vi "RT Acquisition and Logging.vi"(8 "error in (no error)":errorcluster, 10 "info":cluster{"File path":T4, "Cfg ":T5} {"Cfg"."Offset_rueda WS 2" format="%.27g"; "Cfg"."Offset_rueda WS 1" format="%.27g"; "Cfg"."Frecuencia de muestreo y módulo CRIO" items=["51.200 kS/s (NI 9234)"=1, "25.600 kS/s (NI 9234)"=2, "17.067 kS/s (NI 9234)"=3, "12.800 kS/s (NI 9234)"=4, "10.240 kS/s (NI 9234)"=5, "8.533 kS/s (NI 9234)"=6, "7.314 kS/s (NI 9234)"=7, "6.400 kS/s (NI 9234)"=8, "5.689 kS/s (NI 9234)"=9, "5.120 kS/s (NI 9234)"=10, "4.654 kS/s (NI 9234)"=11, "4.267 kS/s (NI 9234)"=12, "3.938 kS/s (NI 9234)"=13, "3.657 kS/s (NI 9234)"=14, "3.413 kS/s (NI 9234)"=15, "3.200 kS/s (NI 9234)"=16, "3.012 kS/s (NI 9234)"=17, "2.845 kS/s (NI 9234)"=18, "2.695 kS/s (NI 9234)"=19, "2.560 kS/s (NI 9234)"=20, "2.438 kS/s (NI 9234)"=21, "2.328 kS/s (NI 9234)"=22, "2.226 kS/s (NI 9234)"=23, "2.133 kS/s (NI 9234)"=24, "2.048 kS/s (NI 9234)"=25, "1.969 kS/s (NI 9234)"=26, "1.896 kS/s (NI 9234)"=27, "1.829 kS/s (NI 9234)"=28, "1.765 kS/s (NI 9234)"=29, "1.707 kS/s (NI 9234)"=30, "1.652 kS/s (NI 9234)"=31]}, 11 "Message Queues in":T7) -> (0 "error out":errorcluster)   [LabVIEW 2015]
uses:
  support/Message Queue/All Message Queues.ctl
  support/Message Queue/Message Cluster.ctl
  controls/File paths.ctl
  controls/Cfg_parameters.ctl
  <vilib>/LabVIEW Targets/FPGA/cRIO/shared/nicrio_ModuleControls/nicrio_cRIO-9234_DataRatesRing2.ctl
  controls/Test Data.ctl
  controls/Acquisition State.ctl
  <vilib>/userdefined/High Color/nirio_resource_hc.ctl
  <vilib>/Platform/TimedLoop/XDataNode/timing_clust.ctl
  <vilib>/Platform/TimedLoop/XDataNode/nitl_modes.ctl
  <vilib>/Platform/TimedLoop/XDataNode/wakeup.ctl
  <vilib>/FPGAPlugInAG/cRIO-9031/niLvFpga_Open_cRIO-9031.vi
  <vilib>/FPGAPlugInAG/cRIO-9031/niLvFpga_Run_cRIO-9031.vi
  <vilib>/Utility/error.llb/Error Cluster From Error Code.vi
  <vilib>/rvi/errors/niLvFpgaAdjustHostInterfaceError.vi
  support/Message Queue/Enqueue Message (Single).vi
  <vilib>/rvi/interface/common/niFpgaWaitOnOcc.vi
  <vilib>/FPGAPlugInAG/cRIO-9031/niLvFpga_Reset_cRIO-9031.vi
  <vilib>/FPGAPlugInAG/cRIO-9031/niLvFpga_Close_cRIO-9031.vi
  <vilib>/rvi/interface/nirviOpenFPGA/nirviOpenFPGA.xnode
  FPGA Bitfiles/W&RDArabia_FPGATarget_FPGA8a2wsBIdirec_yJvL9yuTbZw.lvbitx
  <vilib>/rvi/interface/nirviMethod/nirviMethod.xnode
  <vilib>/rvi/interface/nirviReadWriteControl/nirviReadWriteControl.xnode
  <vilib>/platform/TimedLoop/XDataNode/XDataNode.xnode
  <vilib>/rvi/interface/nirviCloseFPGA/nirviCloseFPGA.xnode
  <vilib>/ErrorRing/Error Ring.xnode
  support/Message Queue/Message Queue.lvlib
  NiFpgaLv.dll
  <vilib>/Platform/TimedLoop/XDataNode/XDNodeRunTimeDep.lvlib
  <vilib>/rvi/errors/niLvFpgaMergeErrorWithErrorCode.vi
  <vilib>/FPGAPlugInAG/cRIO-9031/niLvFpga_ConfigureFifo_cRIO-9031.vi
  <vilib>/FPGAPlugInAG/cRIO-9031/niLvFpga_StartFifo_cRIO-9031.vi
  <vilib>/FPGAPlugInAG/cRIO-9031/niLvFpga_ReadFifo_cRIO-9031.vi
  <vilib>/FPGAPlugInAG/cRIO-9031/niLvFpga_StopFifo_cRIO-9031.vi
panel:
  out "result":bool
  in  "Calibration":T1
  out "Adquirir manual":bool
  out "Tiempo":dbl
  out "Reset_controlador":bool
  in  "trigger":T2
  in  "Test":T3
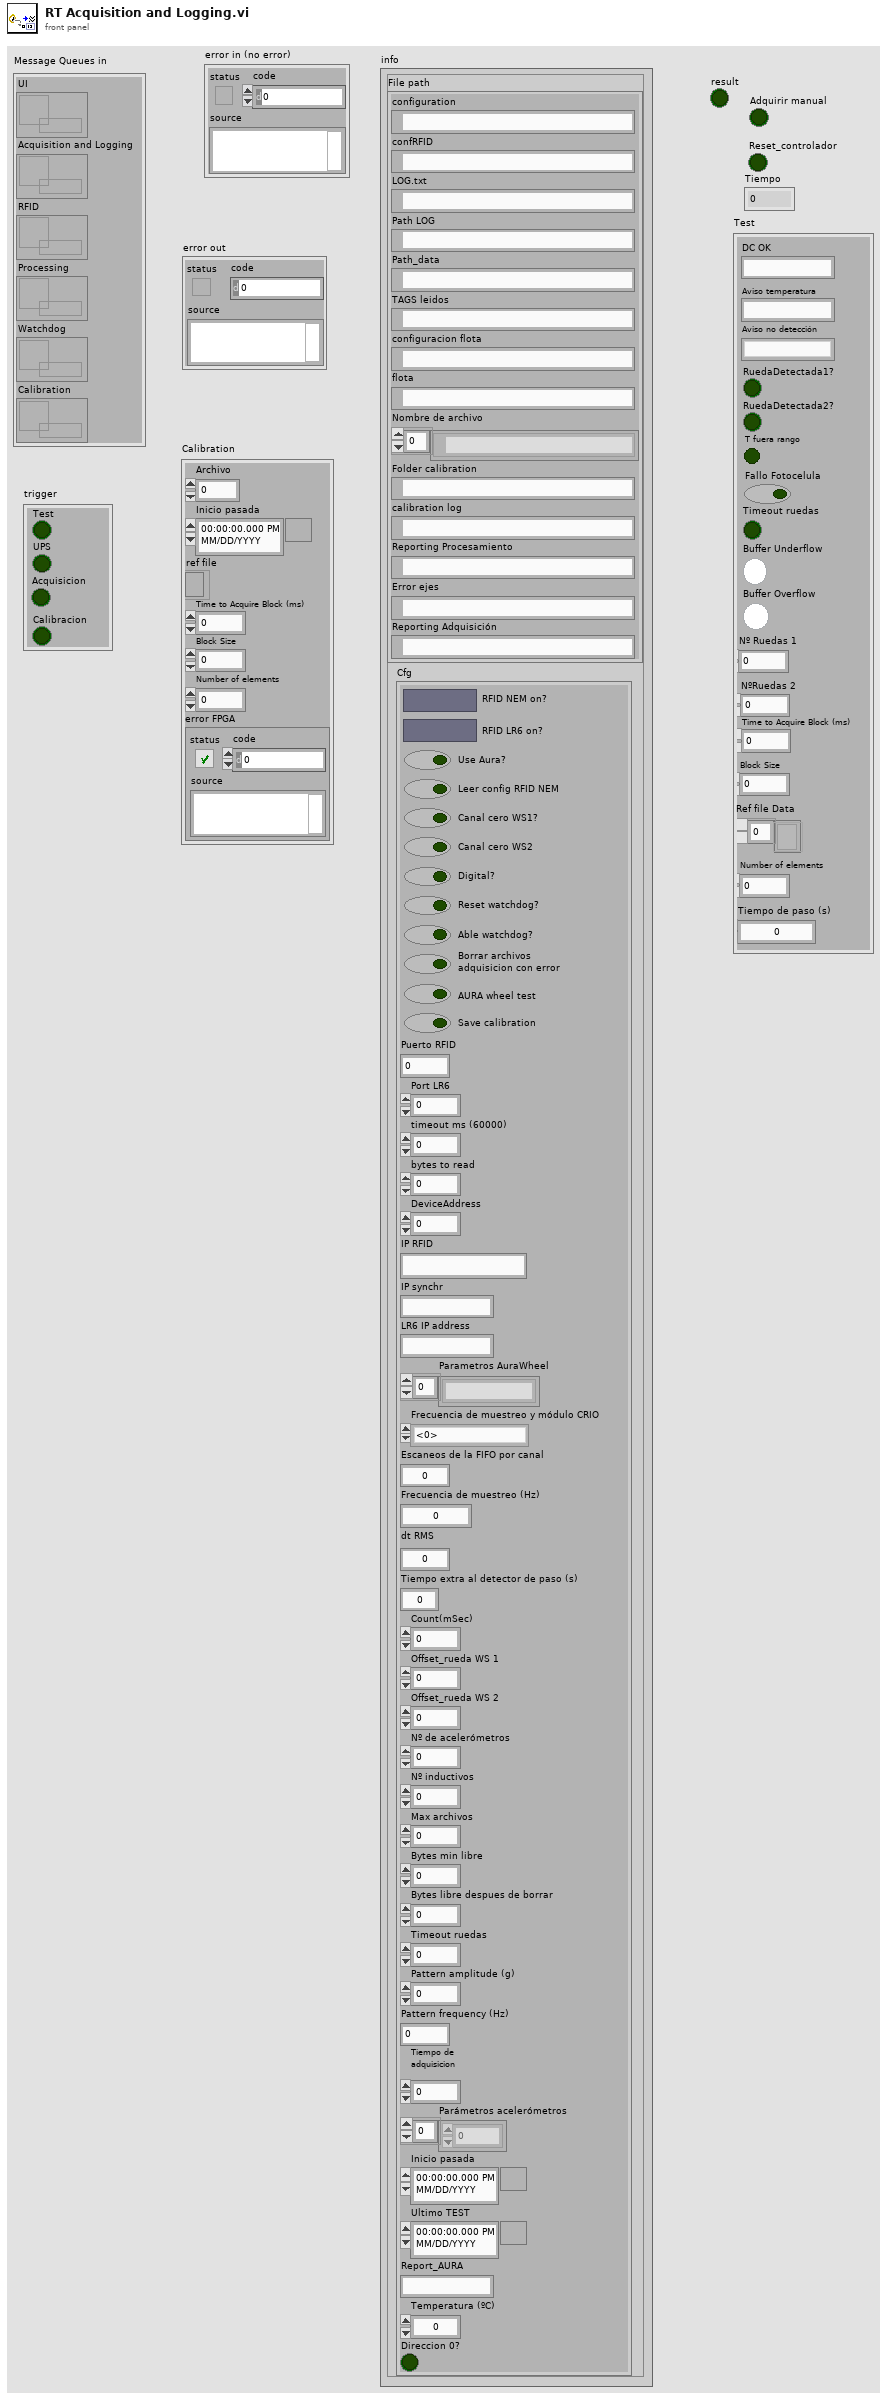
[diagram p1: front panel]
types:
  T1 = cluster{"Archivo":dbl, "Inicio pasada ":timestamp, "ref file":refnum<file>, "Time to Acquire Block (ms)":i32, "Block Size":u32, "Number of elements":u32, "error FPGA":errorcluster}
  T2 = cluster{"Test":bool, "UPS":bool, "Acquisicion":bool, "Calibracion":bool}
  T3 = typedef "Test Data.ctl" = cluster{"DC OK":string, "Aviso temperatura":string, "Aviso no detección":string, "RuedaDetectada1?":bool, "RuedaDetectada2?":bool, "T fuera rango":bool, "Fallo Fotocelula":bool, "Timeout ruedas":bool, "Buffer Underflow":bool, "Buffer Overflow":bool, "Nº Ruedas 1":i32, "NºRuedas 2":i32, "Block Size":u32, "Time to Acquire Block (ms)":i32, "Ref file Data":refnum<file>[], "Number of elements":u32, "Tiempo de paso (s)":dbl}
  T4 = typedef "File paths.ctl" = cluster{"configuration":path, "confRFID":path, "LOG.txt":path, "Path LOG":path, "Path_data":path, "TAGS leidos":path, "configuracion flota":path, "flota":path, "Nombre de archivo":path[], "Folder calibration":path, "calibration log":path, "Reporting Procesamiento":path, "Error ejes":path, "Reporting Adquisición":path}
  T5 = typedef "Cfg_parameters.ctl" = cluster{"RFID NEM on?":bool, "RFID LR6 on?":bool, "Use Aura?":bool, "Leer config RFID NEM":bool, "Canal cero WS1?":bool, "Canal cero WS2 ":bool, "Digital?":bool, "Reset watchdog?":bool, "Able watchdog?":bool, "Borrar archivos\nadquisicion con error":bool, "AURA wheel test":bool, "Save calibration":bool, "Puerto RFID":u16, "Port LR6":u16, "timeout ms (60000)":i32, "bytes to read":i32, "DeviceAddress":u8, "IP RFID":string, "IP synchr":string, "LR6 IP address":string, "Parametros AuraWheel":string[], "Frecuencia de muestreo y módulo CRIO":T6, "Escaneos de la FIFO por canal":u32, "Frecuencia de muestreo (Hz)":dbl, "dt RMS":dbl, "Tiempo extra al detector de paso (s)":dbl, "Count(mSec)":u32, "Offset_rueda WS 1":fxp<+/-,24,-4>, "Offset_rueda WS 2":fxp<+/-,24,-4>, "Nº de acelerómetros":i32, "Nº inductivos":i32, "Max archivos":u32, "Bytes min libre":u32, "Bytes libre despues de borrar":u32, "Timeout ruedas":dbl, "Pattern amplitude (g)":dbl, "Pattern frequency (Hz)":dbl, "Tiempo de adquisicion\n":dbl, "Parámetros acelerómetros":dbl[], "Inicio pasada":timestamp, "Ultimo TEST":timestamp, "Report_AURA":string, "Temperatura (ºC)":dbl, "Direccion 0?":bool}
  T6 = typedef "nicrio_cRIO-9234_DataRatesRing2.ctl" = u8
  T7 = typedef "Message Queue.lvlib/All Message Queues.ctl" = cluster{"UI":refnum<queue>, "Acquisition and Logging":refnum<queue>, "RFID":refnum<queue>, "Processing":refnum<queue>, "Watchdog":refnum<queue>, "Calibration":refnum<queue>}
  T8 = typedef "Acquisition State.ctl" = enum16{"Idle", "Waiting_trigger", "Acquiring", "Calibration", "Calibration_acq"}
  T9 = typedef "nirio_resource_hc.ctl" = tag
  T10 = enum16{"open", "replace", "create", "open or create", "replace or create", "replace or create with confirmation"}
  T11 = typedef "XDNodeRunTimeDep.lvlib/timing_clust.ctl" = cluster{"Expected End [f-1]":u64, "Actual End [f-1]":u64, "Finished Late? [f-1]":bool, "Expected End [i-1]":u64, "Actual End [i-1]":u64, "Finished Late? [i-1]":bool, "Expected Start [i]":u64, "Actual Start [i]":u64, "Expected Start [f]":u64, "Actual Start [f]":u64, "Source Name":string, "Structure Name":string, "Period":i64, "Deadline":i64, "Offset":i64, "Start":i64, "Priority":i32, "Timeout":i32, "Mode":T12, "Wakeup Reason":T13, "Error":errorcluster, "Source Type":string, "Secondary Source Type":string, "Global End Time":u64, "Global Start Time":u64, "Frame Duration":u64, "Iteration Duration":u64, "Assigned CPU":i32, "I/O Scan Engine Mode":u32}
  T12 = typedef "XDNodeRunTimeDep.lvlib/nitl_modes.ctl" = enum32{"No Change", "Process missed periods, maintain original phase", "Discard missed periods, maintain original phase", "Process missed periods, ignore original phase", "Discard missed periods, ignore original phase"}
  T13 = typedef "XDNodeRunTimeDep.lvlib/wakeup.ctl" = enum32{"Normal", "Aborted", "Asynchronous wakeup", "Timing source error", "Timed loop error", "Timeout"}
  T14 = cluster{"error IO":errorcluster, dbl[], "Direccion 0?":bool, "error out":errorcluster}
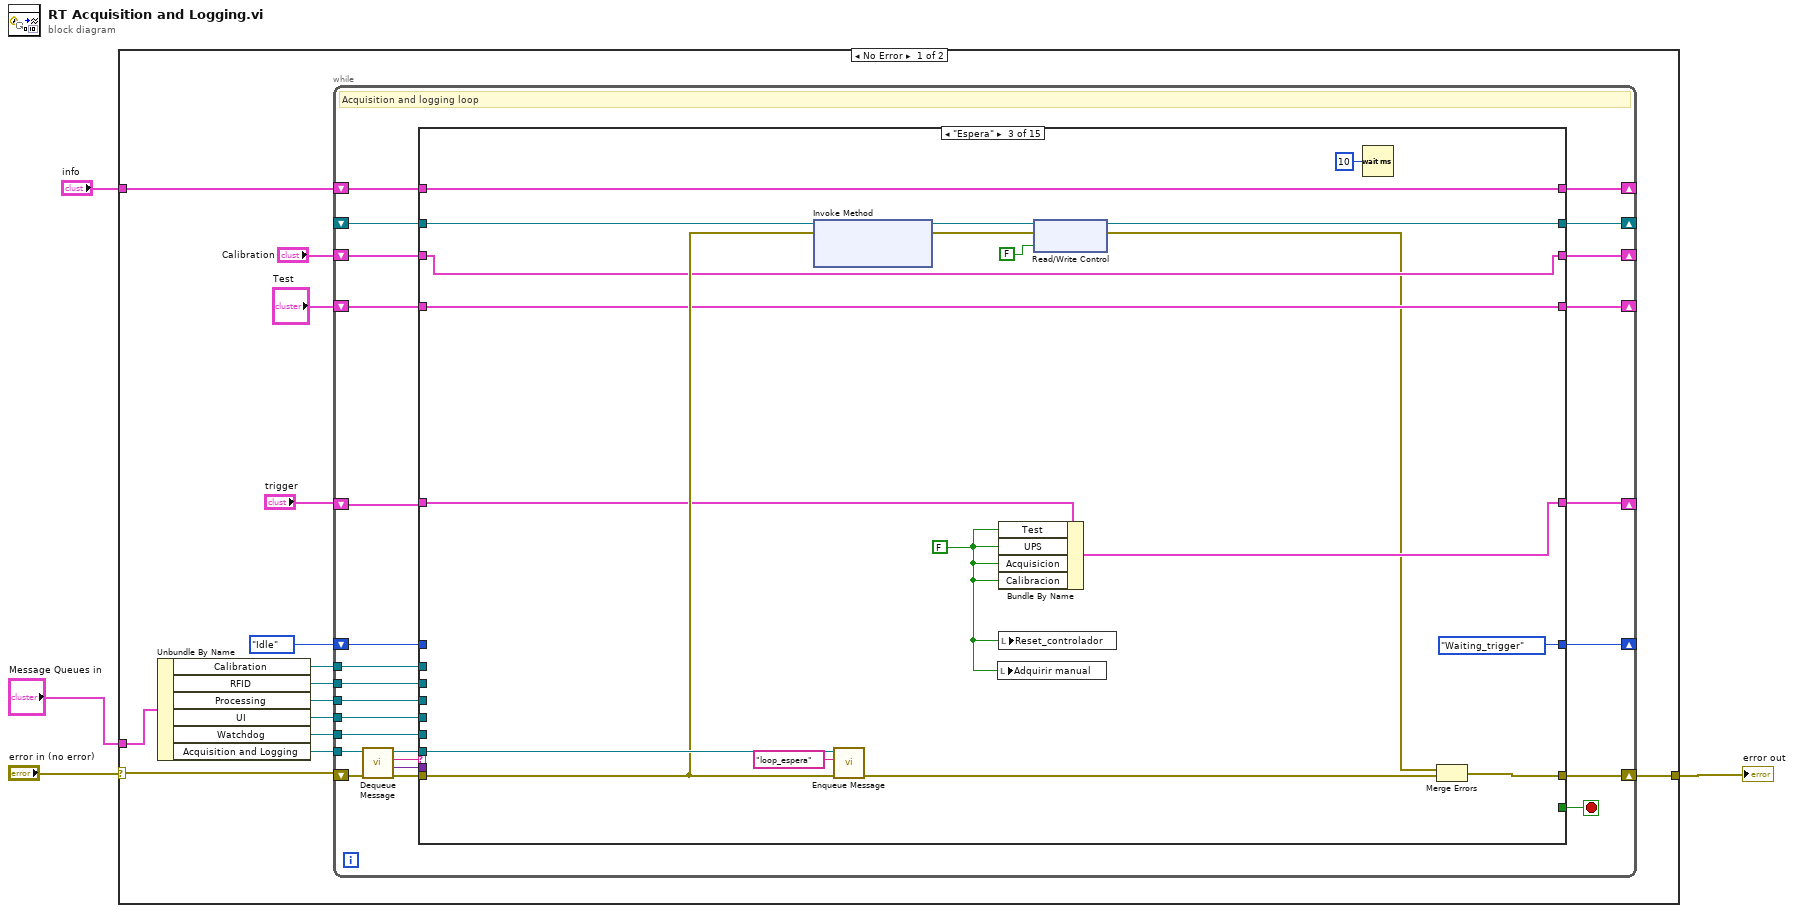
[diagram p0: block diagram]
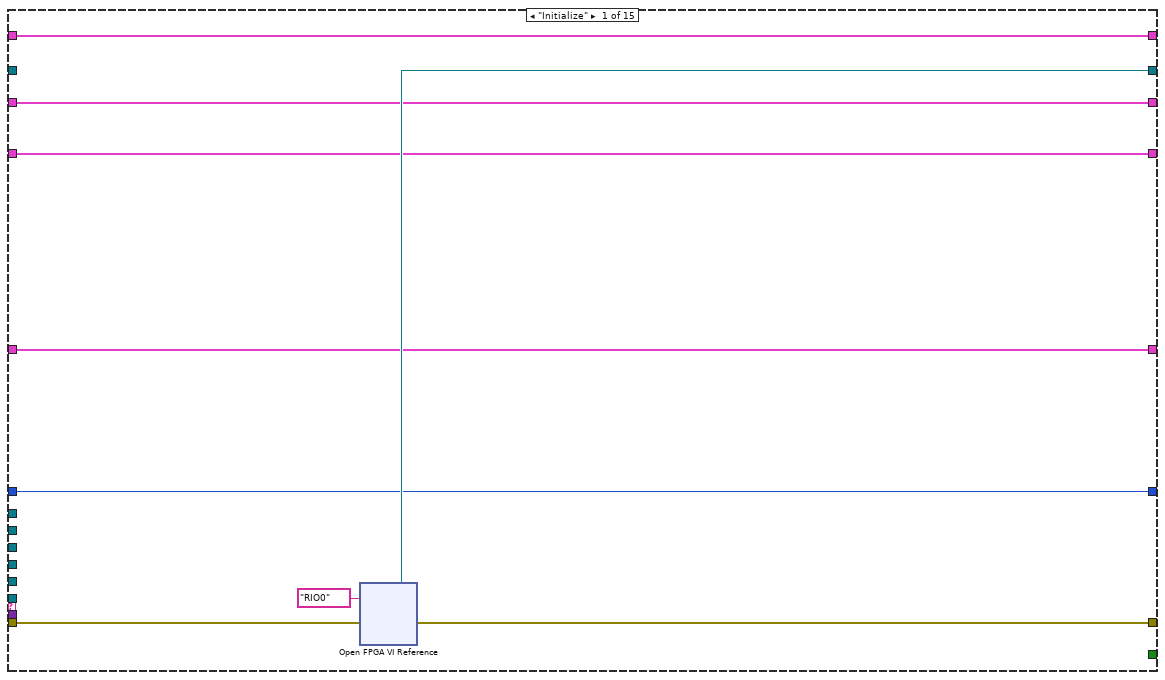
[diagram p2: hidden frame]
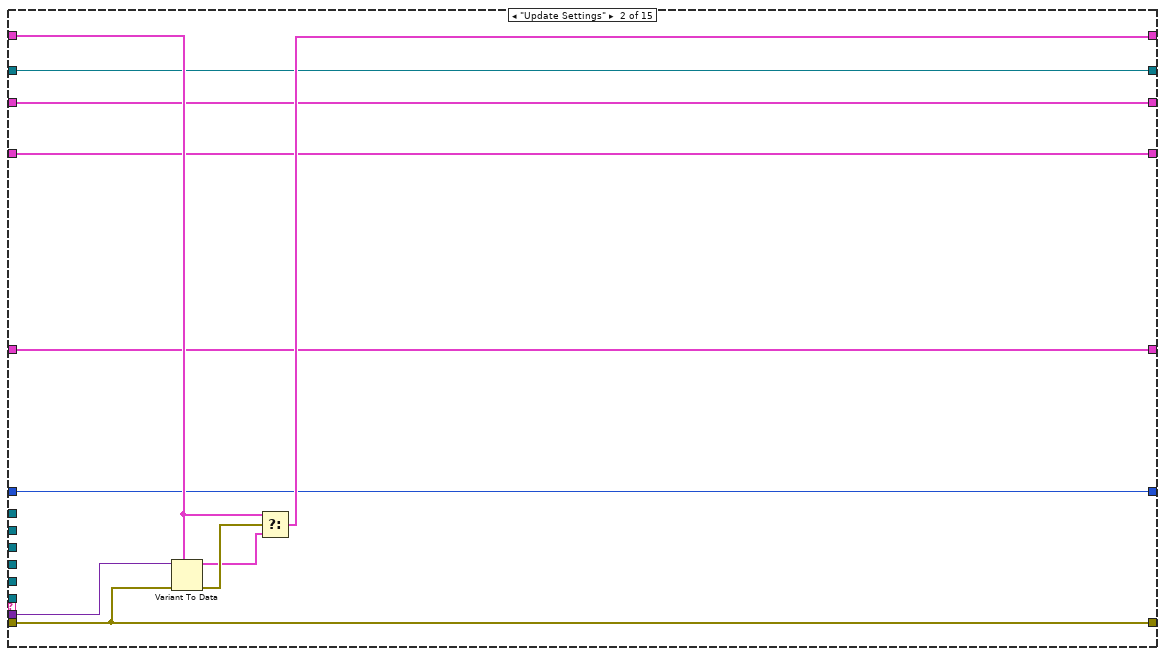
[diagram p3: hidden frame]
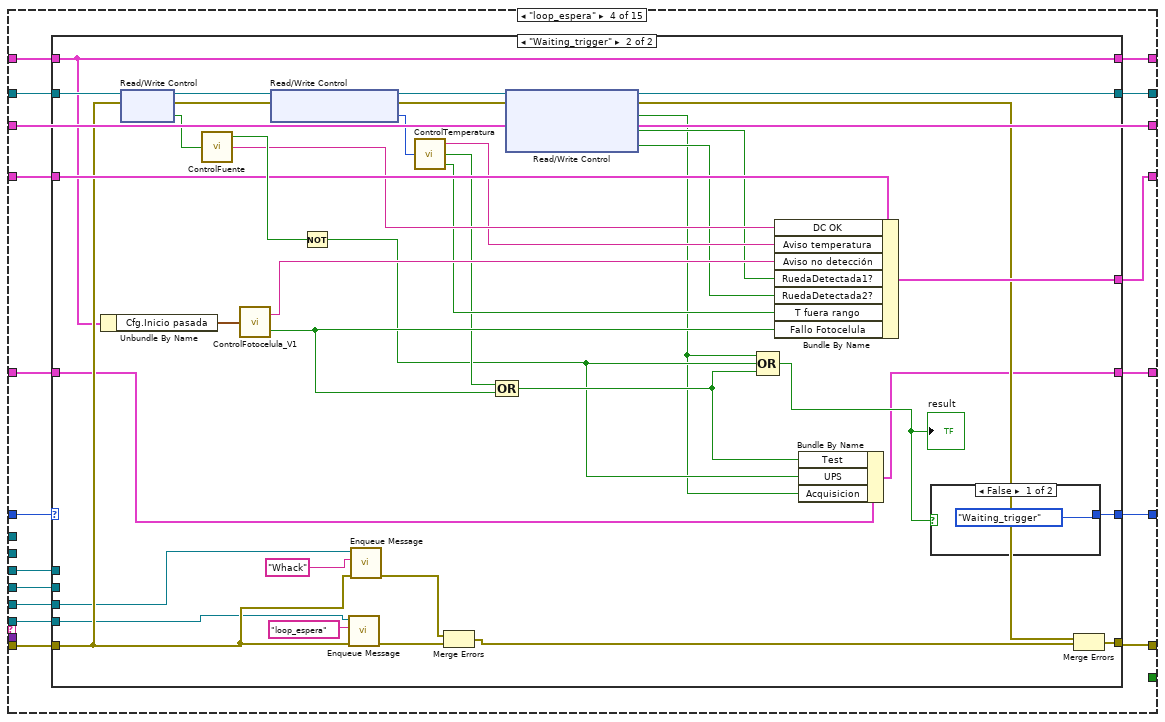
[diagram p4: hidden frame]
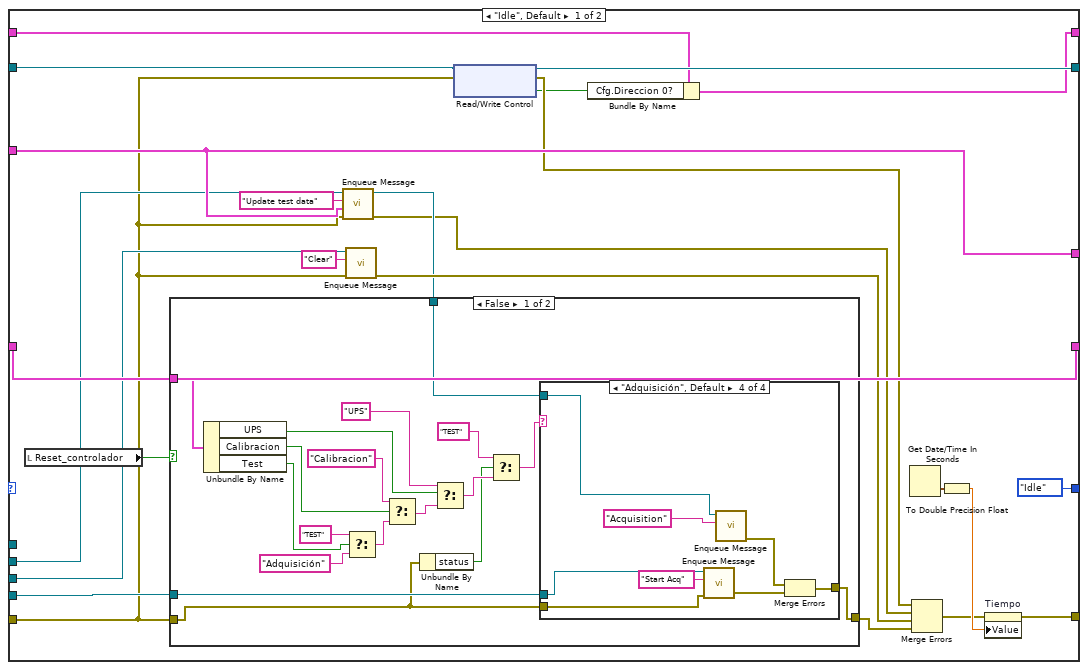
[diagram p5: hidden frame]
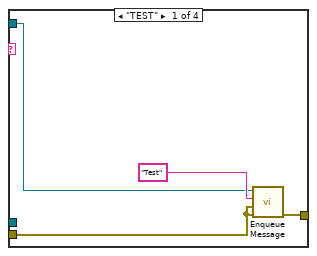
[diagram p6: hidden frame]
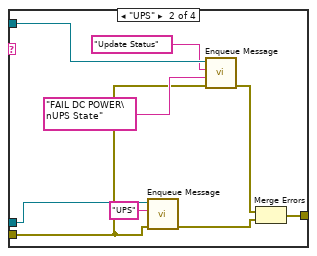
[diagram p7: hidden frame]
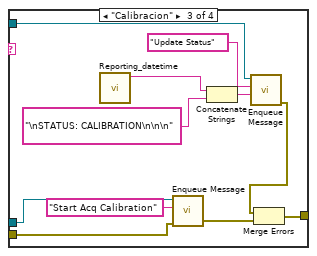
[diagram p8: hidden frame]
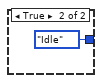
[diagram p10: hidden frame]
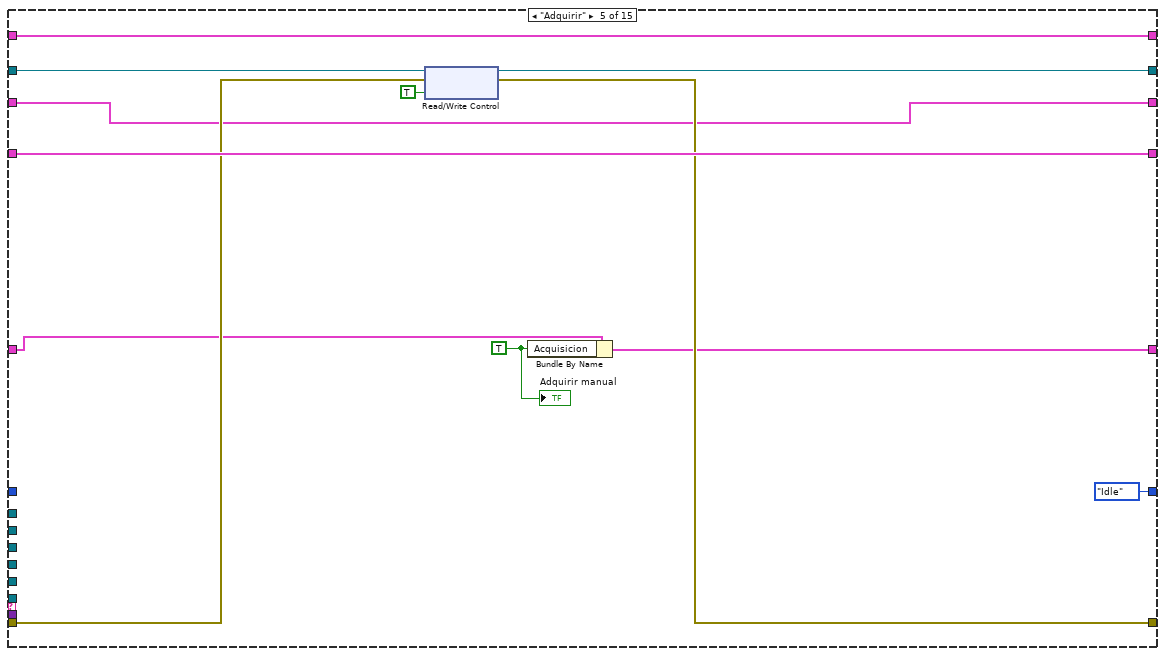
[diagram p11: hidden frame]
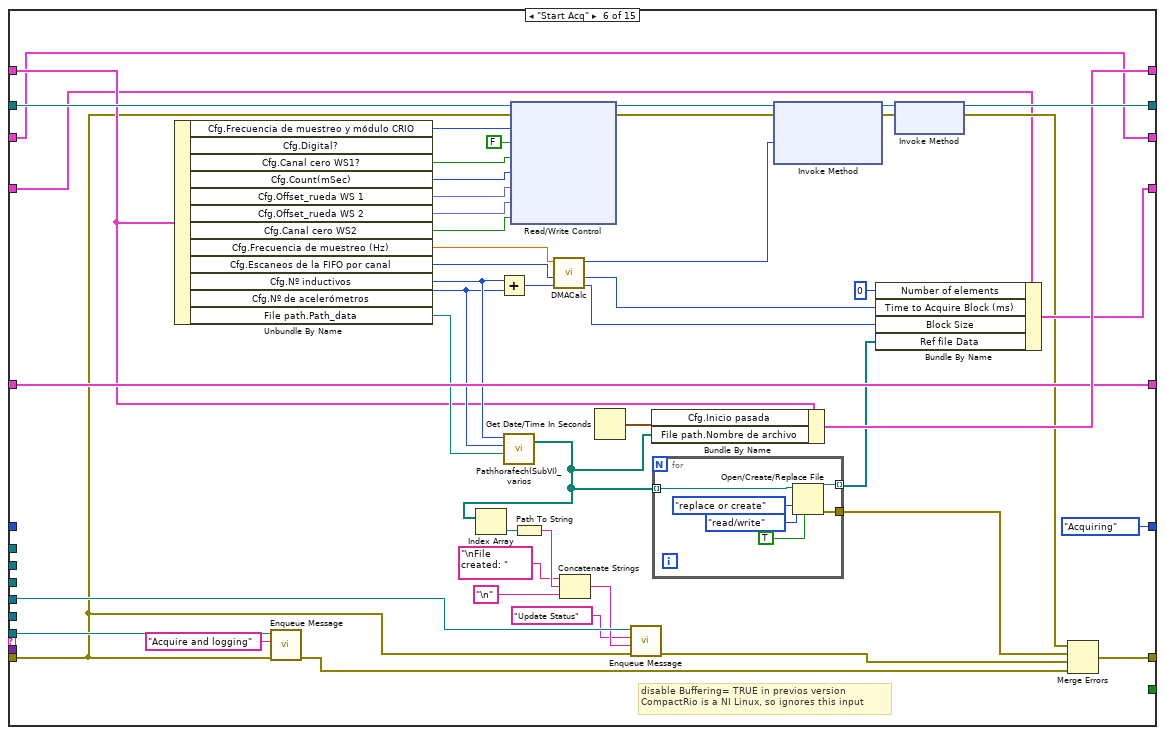
[diagram p12: hidden frame]
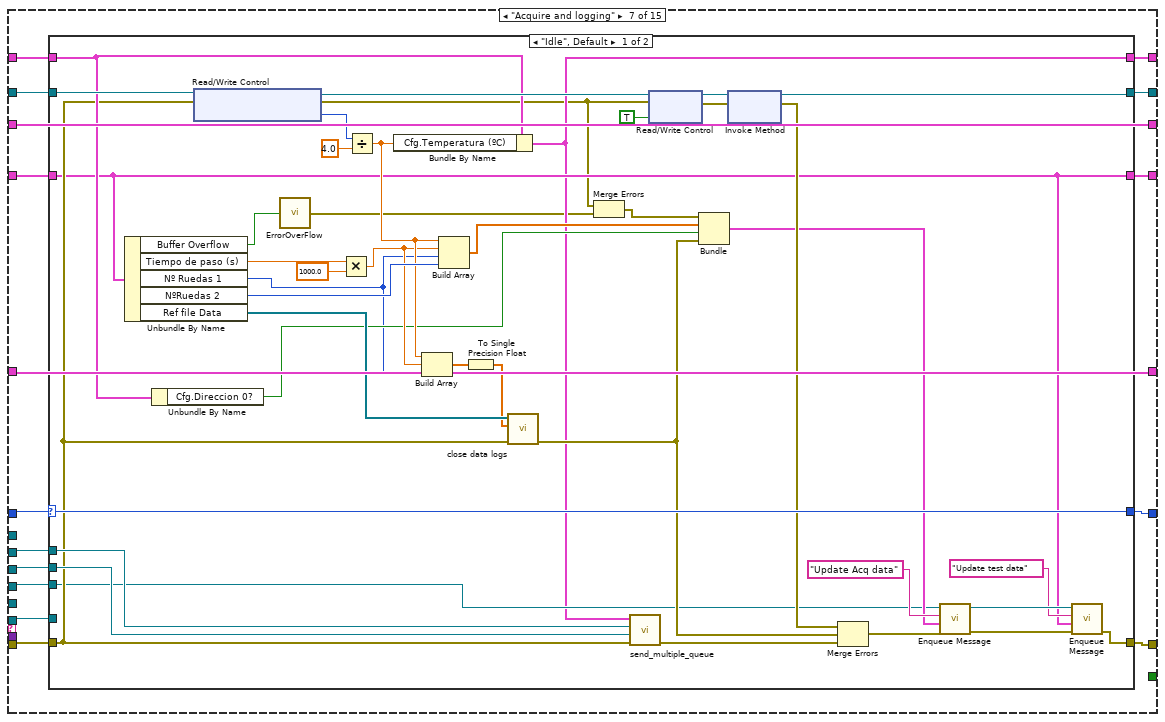
[diagram p13: hidden frame]
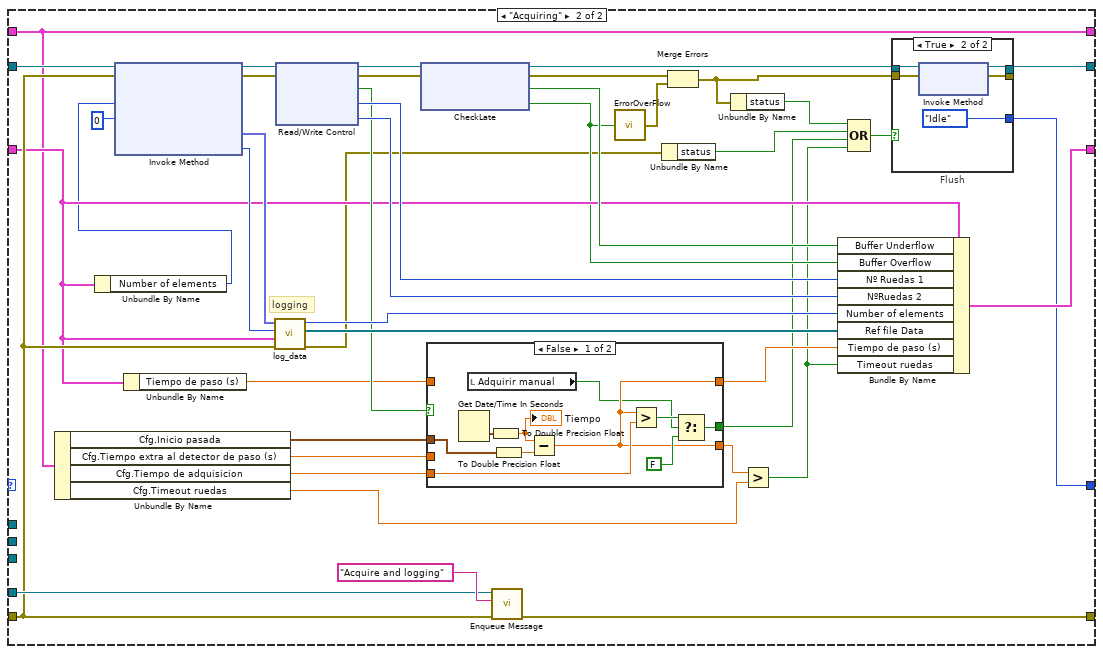
[diagram p14: hidden frame]
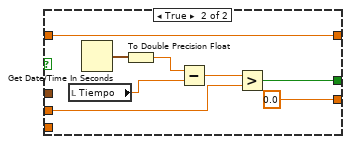
[diagram p15: hidden frame]
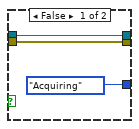
[diagram p16: hidden frame]
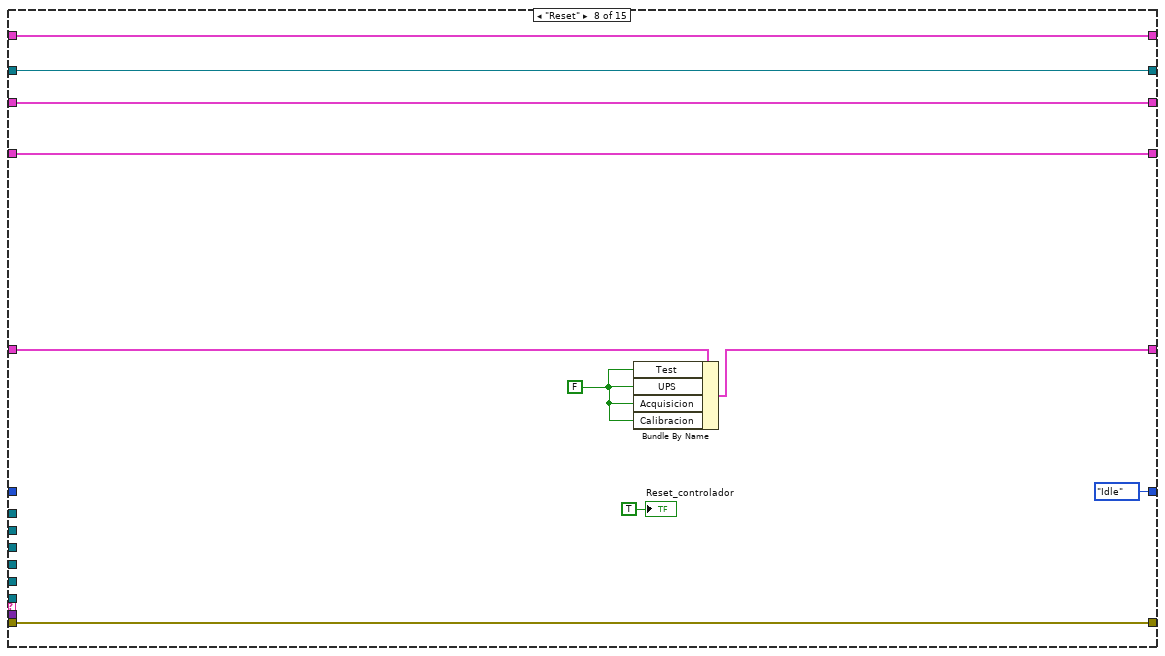
[diagram p17: hidden frame]
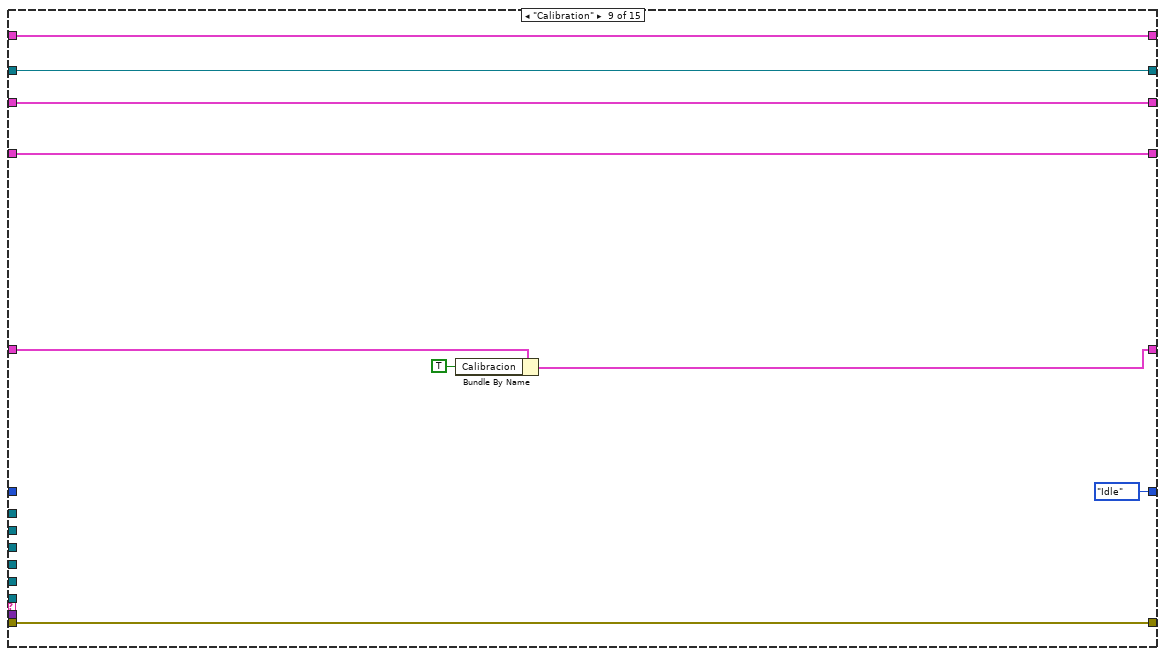
[diagram p18: hidden frame]
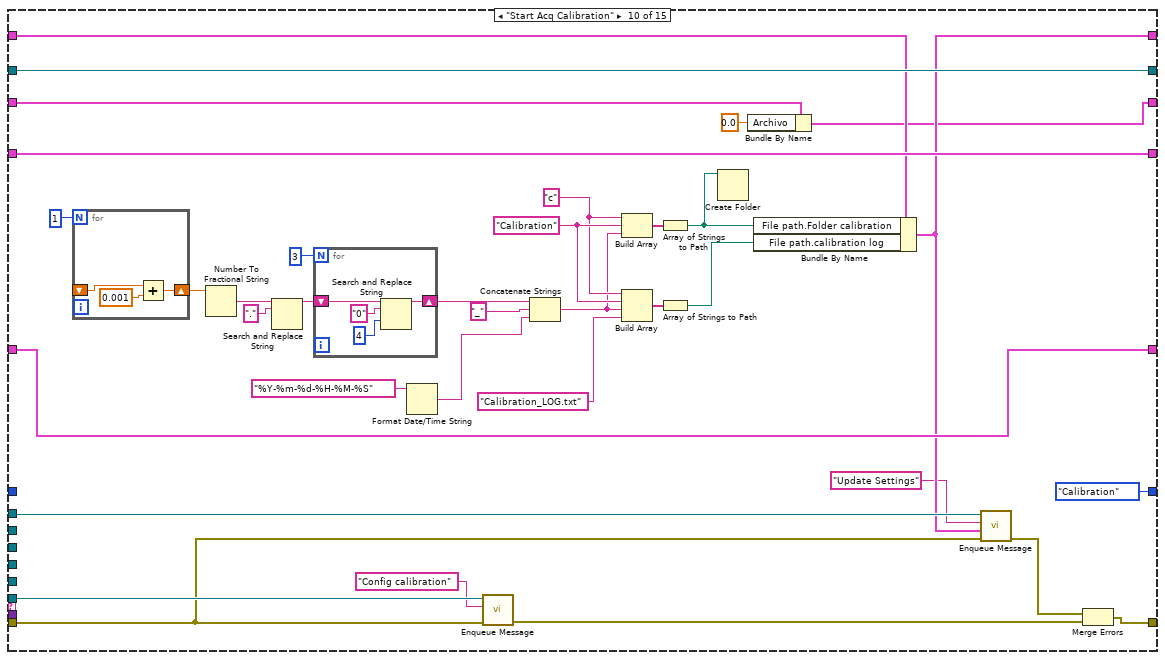
[diagram p19: hidden frame]
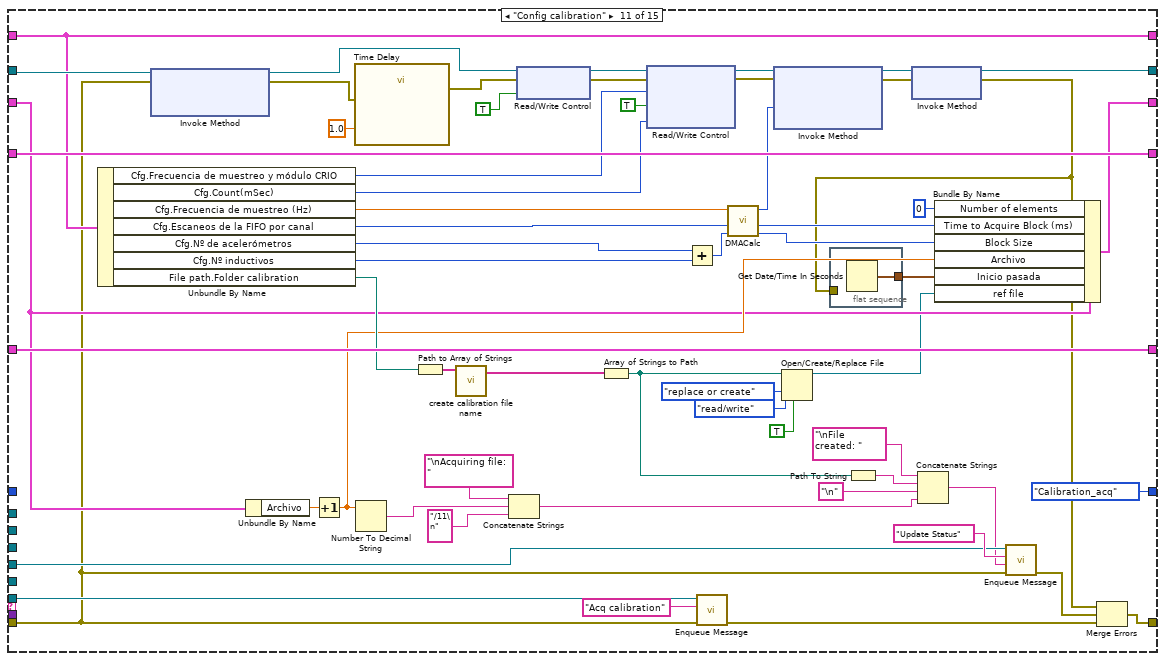
[diagram p20: hidden frame]
diagram:
  n1 = case shown="No Error" "error in (no error)" {
    selector: "error in (no error)" -> [w17 w679]
    tunnel: "Message Queues in" -> [w18 _]
    tunnel: "info" -> [w14 _]
    tunnel: [w13 w679] -> w1
    frame No Error {
      n2 = Unbundle By Name(w18) -> ("Calibration"=w6:refnum<queue>, "RFID"=w7:refnum<queue>, "Processing"=w8:refnum<queue>, "UI"=w11:refnum<queue>, "Watchdog"=w15:refnum<queue>, "Acquisition and Logging"=w16:refnum<queue>)
      n3 = while {
        tunnel: w16 -> [w42]
        tunnel: w15 -> [w40]
        shift-right: [w36] -> _
        shift-left: w14 -> [w37]
        shift-right: [w32] -> _
        shift-left: _ -> [w31]
        shift-right: [w29] -> _
        shift-left: Acquisition_State."Idle" ("Acquisition State") -> [w30]
        tunnel: w11 -> [w28]
        shift-right: [w26] -> _
        shift-left: "Test" -> [w27]
        shift-right: [w34] -> w13
        shift-left: w17 -> [w43]
        shift-right: [w24] -> _
        shift-left: "trigger" -> [w25]
        tunnel: w8 -> [w23]
        tunnel: w7 -> [w22]
        tunnel: w6 -> [w21]
        shift-right: [w19] -> _
        shift-left: "Calibration" -> [w20]
        stop <- w35 stop-if-true
        # "Acquisition and logging loop"
        n4 = call "Dequeue Message.vi"("error in (no error)"=w43, "Message Queue"=w42) -> ("error out"=w39:errorcluster, "Message Data"=w33:variant, "Message"=w38:string, "dup Message Queue"=w41:refnum<queue>)  [unwired: 6 in]
        n5 = case shown="\"Espera\"" w38 {
          selector: w38 -> [_ _ _ _ _ _ _ _ _ _ _ _ _ _ w669]
          tunnel: w41 -> [_ _ w79 w93 _ w251 w290 _ _ w436 w491 w530 _ w661 _]
          tunnel: w40 -> [_ _ _ w92 _ _ _ _ _ _ _ _ _ _ _]
          tunnel: w39 -> [w50 w60 w77 w94 w221 w230 w293 w411 w417 w433 w467 w534 w634 w662 _]
          tunnel: [w49 w60 w76 w95 w220 w237 w288 w411 w417 w432 w473 w531 w629 w658 w670] -> w34
          tunnel: w37 -> [w52 w59 w82 w86 w223 w231 w287 w415 w424 w440 w505 w528 w639 w663 w671]
          tunnel: [w52 w58 w82 w85 w223 w260 w285 w415 w424 w434 w505 w528 w639 w663 w671] -> w36
          tunnel: [_ _ _ _ _ _ _ _ _ _ _ _ _ TRUE _] -> w35
          tunnel: w33 -> [_ w63 _ _ _ _ _ _ _ _ _ _ _ _ _]
          tunnel: [w48 w57 w64 w98 w224 w268 w282 w413 w423 w459 w506 w537 w635 _ w668] -> w32
          tunnel: w31 -> [_ w57 w81 w99 w226 w269 w295 w413 w423 w459 w522 w540 w636 w657 w668]
          tunnel: w30 -> [w47 w56 _ w91 _ _ w296 _ _ _ _ w541 _ _ w667]
          tunnel: [w47 w56 Acquisition_State."Waiting_trigger" ("Acquisition State") w83 Acquisition_State."Idle" ("Acquisition State") Acquisition_State."Acquiring" ("Acquisition State") w291 Acquisition_State."Idle" ("Acquisition State") Acquisition_State."Idle" ("Acquisition State") Acquisition_State."Calibration" ("Acquisition State") Acquisition_State."Calibration_acq" ("Acquisition State") w532 Acquisition_State."Idle" ("Acquisition State") Acquisition_State."Idle" ("Acquisition State") w667] -> w29
          tunnel: w28 -> [_ _ _ w88 _ w242 w283 _ _ _ w480 w529 w628 _ _]
          tunnel: w27 -> [w46 w55 w74 w97 w222 w229 w294 w414 w422 w458 w525 w536 w633 w655 w666]
          tunnel: [w46 w55 w74 w96 w222 w252 w289 w414 w422 w458 w525 w535 w633 w655 w666] -> w26
          tunnel: w25 -> [w45 w54 w73 w90 w218 w255 w292 w410 w421 w437 w524 w539 w631 w654 w665]
          tunnel: [w45 w54 w72 w89 w217 w255 w292 w409 w420 w437 w524 w539 w631 w654 w665] -> w24
          tunnel: w23 -> [_ _ _ w87 _ _ w284 _ _ _ _ _ _ _ _]
          tunnel: w22 -> [_ _ _ _ _ _ w286 _ _ _ _ _ _ _ _]
          tunnel: w21 -> [_ _ _ _ _ _ _ _ _ w435 _ w527 _ _ _]
          tunnel: [w44 w53 w70 w84 w215 w228 w281 w406 w416 w425 w494 w533 w626 w653 w664] -> w19
          tunnel: w20 -> [w44 w53 w70 w84 w215 w228 w281 w406 w416 w427 w488 w538 w626 w653 w664]
          frame "Initialize" {
            n6 = xnode "Open FPGA VI Reference"("error in"=w50, "resource name"=T9 "RIO0") -> ("FPGA VI Reference Out"=w48:refnum<k20>, "error out"=w49:errorcluster)
          }
          frame "Update Settings" {
            n7 = Variant To Data(error in=w60, type=w59, Variant=w63) -> (data=w61:cluster{"File path":T4, "Cfg ":T5}, error out=w62:errorcluster)
            n8 = Select(t=w59, s=w62, f=w61) -> (s? t:f=w58:cluster{"File path":T4, "Cfg ":T5})
          }
          frame "Espera" {
            w71 = FALSE ("Test")
            n9 = xnode "Invoke Method"("FPGA VI Reference In"=w81, "error in"=w77) -> ("FPGA VI Reference Out"=w65:refnum<k20>, "error out"=w67:errorcluster)  [unwired: 1 in]
            n10 = call-poly "Enqueue Message.vi"("error in (no error)"=w77, "Message"="loop_espera", "Message Queue"=w79) -> ("error out"=w75:errorcluster)  [unwired: 7 in, 1 out]
            n11 = local write "Adquirir manual"(w71) -> ()
            n12 = Bundle By Name(cluster=w73, "Test"=w71, "UPS"=w71, "Acquisicion"=w71, "Calibracion"=w71) -> (w72:T2)
            n13 = local write "Reset_controlador"(w71) -> ()
            n14 = xnode "Read/Write Control"("FPGA VI Reference In"=w65, "error in"=w67, "Fotocélula"=FALSE) -> ("FPGA VI Reference Out"=w64:refnum<k20>, "error out"=w66:errorcluster)
            n15 = Wait (ms)(milliseconds to wait=u32 10) -> ()  [unwired: 1 out]
            n16 = Merge Errors(w66, w75) -> (w76:errorcluster)
          }
          frame "loop_espera" {
            n17 = case shown="\"Waiting_trigger\"" w91 {
              tunnel: w99 -> [w113 w208]
              tunnel: [w114 w207] -> w98
              tunnel: w86 -> [w104 w176]
              tunnel: w97 -> [w117 w202]
              tunnel: [w117 w201] -> w96
              tunnel: [Acquisition_State."Idle" ("Acquisition State") w192] -> w83
              tunnel: [w108 w190] -> w95
              tunnel: w94 -> [w110 w189]
              tunnel: w93 -> [w111 w187]
              tunnel: w92 -> [w120 w186]
              tunnel: w90 -> [w122 w181]
              tunnel: [w122 w177] -> w89
              tunnel: w88 -> [w112 _]
              tunnel: w87 -> [_ _]
              tunnel: [w103 w176] -> w85
              frame "Idle", Default {
                n18 = local read "Reset_controlador"() -> (w121:bool)
                n19 = call-poly "Enqueue Message.vi"("error in (no error)"=w110, "Message Data"=w117, "Message"="Update test data", "Message Queue"=w112) -> ("error out"=w100:errorcluster, "dup Message Queue"=w101:refnum<queue>)  [unwired: 6 in]
                n20 = case shown="False" w121 {
                  tunnel: w122 -> [w141 _]
                  tunnel: w111 -> [w130 _]
                  tunnel: w101 -> [w134 _]
                  tunnel: w110 -> [w125 w174]
                  tunnel: [w129 w174] -> w106
                  frame False {
                    n21 = Unbundle By Name(w141) -> ("UPS"=w135:bool, "Calibracion"=w133:bool, "Test"=w131:bool)
                    n22 = Select(t="TEST", s=w131, f="Adquisición") -> (s? t:f=w132:string)
                    n23 = Select(t="Calibracion", s=w133, f=w132) -> (s? t:f=w139:string)
                    n24 = Unbundle By Name(w125) -> ("status"=w124:bool)
                    n25 = Select(t="UPS", s=w135, f=w139) -> (s? t:f=w128:string)
                    n26 = Select(t="TEST", s=w124, f=w128) -> (s? t:f=w126:string)
                    n27 = case shown="\"Adquisición\", Default" w126 {
                      tunnel: w134 -> [w144 w154 w161 w166]
                      tunnel: w130 -> [_ w153 w156 w168]
                      tunnel: w125 -> [w142 w151 w157 w169]
                      tunnel: [w143 w147 w160 w172] -> w129
                      frame "TEST" {
                        n28 = call-poly "Enqueue Message.vi"("error in (no error)"=w142, "Message Data"=w142, "Message"="Test", "Message Queue"=w144) -> ("error out"=w143:errorcluster)  [unwired: 6 in, 1 out]
                      }
                      frame "UPS" {
                        n29 = call-poly "Enqueue Message.vi"("error in (no error)"=w151, "Message"="UPS", "Message Queue"=w153) -> ("error out"=w148:errorcluster)  [unwired: 7 in, 1 out]
                        n30 = call-poly "Enqueue Message.vi"("error in (no error)"=w151, "Message Data"="FAIL DC POWER\nUPS State", "Message"="Update Status", "Message Queue"=w154) -> ("error out"=w149:errorcluster)  [unwired: 6 in, 1 out]
                        n31 = Merge Errors(w149, w148) -> (w147:errorcluster)
                      }
                      frame "Calibracion" {
                        n32 = call "Reporting_datetime.vi"() -> ("String"=w164:string)  [unwired: 11 in]
                        n33 = call-poly "Enqueue Message.vi"("error in (no error)"=w157, "Message"="Start Acq Calibration", "Message Queue"=w156) -> ("error out"=w158:errorcluster)  [unwired: 7 in, 1 out]
                        n34 = Concatenate Strings(w164, "\nSTATUS: CALIBRATION\n\n\n") -> (w165:string)
                        n35 = call-poly "Enqueue Message.vi"("Message Data"=w165, "Message"="Update Status", "Message Queue"=w161) -> ("error out"=w159:errorcluster)  [unwired: 7 in, 1 out]
                        n36 = Merge Errors(w159, w158) -> (w160:errorcluster)
                      }
                      frame "Adquisición", Default {
                        n37 = call-poly "Enqueue Message.vi"("error in (no error)"=w169, "Message"="Start Acq", "Message Queue"=w168) -> ("error out"=w170:errorcluster)  [unwired: 7 in, 1 out]
                        n38 = call-poly "Enqueue Message.vi"("Message"="Acquisition", "Message Queue"=w166) -> ("error out"=w171:errorcluster)  [unwired: 8 in, 1 out]
                        n39 = Merge Errors(w171, w170) -> (w172:errorcluster)
                      }
                    }
                  }
                  frame True {
                  }
                }
                n40 = call-poly "Enqueue Message.vi"("error in (no error)"=w110, "Message"="Clear", "Message Queue"=w120) -> ("error out"=w109:errorcluster)  [unwired: 7 in, 1 out]
                n41 = xnode "Read/Write Control"("FPGA VI Reference In"=w113, "error in"=w110) -> ("FPGA VI Reference Out"=w114:refnum<k20>, "error out"=w105:errorcluster, "Direccion 0?"=w102:bool)
                n42 = Bundle By Name(cluster=w104, "Cfg.Direccion 0?"=w102) -> (w103:cluster{"File path":T4, "Cfg ":T5})
                n43 = Get Date/Time In Seconds() -> (seconds since 1Jan1904=w116:timestamp)
                n44 = Merge Errors(w105, w100, w109, w106) -> (w107:errorcluster)
                n45 = To Double Precision Float(number=w116) -> (double precision float=w115:dbl)
                n46 = property on="Tiempo" class="DigNum (strict)"(error in=w107, "Value"=w115) -> (error out=w108:errorcluster)  [unwired: 1 in, 1 out]
              }
              frame "Waiting_trigger" {
                n47 = Unbundle By Name(w176) -> ("Cfg.Inicio pasada"=w206:timestamp)
                n48 = xnode "Read/Write Control"("FPGA VI Reference In"=w208, "error in"=w189) -> ("FPGA VI Reference Out"=w212:refnum<k20>, "error out"=w211:errorcluster, "DC OK"=w205:bool)
                n49 = call "ControlFuente.vi"("DC OK 3"=w205) -> ("DC OK 2"=w203:bool, "DC OK"=w200:string)  [unwired: 1 out]
                n50 = call "ControlFotocelula_V1.vi"("Tiempo de entrada a espera"=w206) -> ("Aviso no detección"=w198:string, "Boolean"=w194:bool)
                n51 = xnode "Read/Write Control"("FPGA VI Reference In"=w212, "error in"=w211) -> ("FPGA VI Reference Out"=w210:refnum<k20>, "error out"=w209:errorcluster, "Chassis Temperature"=w204:i16)
                n52 = Not(x=w203) -> (.not. x?=w178:bool)
                n53 = call-poly "Enqueue Message.vi"("error in (no error)"=w189, "Message"="loop_espera", "Message Queue"=w187) -> ("error out"=w184:errorcluster)  [unwired: 7 in, 1 out]
                n54 = call-poly "Enqueue Message.vi"("error in (no error)"=w189, "Message"="Whack", "Message Queue"=w186) -> ("error out"=w183:errorcluster)  [unwired: 7 in, 1 out]
                n55 = call "ControlTemperatura.vi"("Chassis Temperature"=w204) -> ("Aviso temperatura"=w199:string, "Boolean"=w193:bool, "T fuera rango"=w195:bool)
                n56 = Merge Errors(w183, w184) -> (w188:errorcluster)
                n57 = Compound Arithmetic op=OR(w193, w194) -> (w180:bool)
                n58 = xnode "Read/Write Control"("FPGA VI Reference In"=w210, "error in"=w209) -> ("FPGA VI Reference Out"=w207:refnum<k20>, "error out"=w191:errorcluster, "Detector de presencia"=w175:bool, "RuedaDetectada1?"=w197:bool, "RuedaDetectada2?"=w196:bool)
                n59 = Compound Arithmetic op=OR(w175, w178, w180) -> (w179:bool)
                "result" <- w179
                n60 = Bundle By Name(cluster=w202, "DC OK"=w200, "Aviso temperatura"=w199, "Aviso no detección"=w198, "RuedaDetectada1?"=w197, "RuedaDetectada2?"=w196, "T fuera rango"=w195, "Fallo Fotocelula"=w194) -> (w201:T3)
                n61 = Bundle By Name(cluster=w181, "Test"=w180, "UPS"=w178, "Acquisicion"=w175) -> (w177:T2)
                n62 = case shown="False" w179 {
                  tunnel: [Acquisition_State."Waiting_trigger" ("Acquisition State") Acquisition_State."Idle" ("Acquisition State")] -> w192
                  frame False {
                  }
                  frame True {
                  }
                }
                n63 = Merge Errors(w191, w188) -> (w190:errorcluster)
              }
            }
          }
          frame "Adquirir" {
            w216 = TRUE ("Acquisicion")
            n64 = xnode "Read/Write Control"("FPGA VI Reference In"=w226, "error in"=w221, "Fotocélula"=TRUE) -> ("FPGA VI Reference Out"=w224:refnum<k20>, "error out"=w220:errorcluster)
            n65 = Bundle By Name(cluster=w218, "Acquisicion"=w216) -> (w217:T2)
            "Adquirir manual" <- w216
          }
          frame "Start Acq" {
            # "disable Buffering= TRUE in previos version\nCompactRio is a NI Linux, so ignores this input"
            n66 = Unbundle By Name(w231) -> ("Cfg.Frecuencia de muestreo y módulo CRIO"=w267:T6, "Cfg.Canal cero WS1?"=w266:bool, "Cfg.Count(mSec)"=w265:u32, "Cfg.Offset_rueda WS 1"=w264:fxp<+/-,24,-4>, "Cfg.Offset_rueda WS 2"=w263:fxp<+/-,24,-4>, "Cfg.Canal cero WS2"=w262:bool, "Cfg.Frecuencia de muestreo (Hz)"=w259:dbl, "Cfg.Escaneos de la FIFO por canal"=w258:u32, "Cfg.Nº inductivos"=w245:i32, "Cfg.Nº de acelerómetros"=w244:i32, "File path.Path_data"=w243:path)  [unwired: 1 out]
            n67 = call-poly "Enqueue Message.vi"("error in (no error)"=w230, "Message"="Acquire and logging", "Message Queue"=w251) -> ("error out"=w234:errorcluster)  [unwired: 7 in, 1 out]
            n68 = Add(x=w245, y=w244) -> (x+y=w257:i32)
            n69 = call "Pathhorafech(SubVI)_varios.vi"("Folder path"=w243, "Nº de acelerómetros"=w244, "Nº inductivos"=w245) -> ("Acel_Paths"=w236:path[])  [unwired: 1 in, 1 out]
            n70 = Index Array(array=w236) -> (element=w248:path)  [unwired: 1 in]
            n71 = xnode "Read/Write Control"("FPGA VI Reference In"=w269, "error in"=w230, "Data Rate"=w267, "Digital?"=FALSE, "Canal cero WS1?"=w266, "Count(mSec)"=w265, "Offset_WS1"=w264, "Offset_WS2"=w263, "Canal cero WS2?"=w262) -> ("FPGA VI Reference Out"=w271:refnum<k20>, "error out"=w270:errorcluster)
            n72 = Path To String(path=w248) -> (string=w249:string)
            n73 = call "DMACalc.vi"("Number of Channels"=w257, "Number of Samples"=w258, "Rate (Hz)"=w259) -> ("Block Size"=w253:u32, "Time to Acquire Block (ms)"=w254:i32, "Host Buffer Size"=w256:u32)  [unwired: 6 in]
            n74 = Concatenate Strings("\nFile created: ", w249, "\n") -> (w241:string)
            n75 = Get Date/Time In Seconds() -> (seconds since 1Jan1904=w261:timestamp)
            n76 = call-poly "Enqueue Message.vi"("error in (no error)"=w230, "Message Data"=w241, "Message"="Update Status", "Message Queue"=w242) -> ("error out"=w238:errorcluster)  [unwired: 6 in, 1 out]
            n77 = Bundle By Name(cluster=w231, "Cfg.Inicio pasada"=w261, "File path.Nombre de archivo"=w236) -> (w260:cluster{"File path":T4, "Cfg ":T5})
            n78 = for {
              tunnel: w236 -> [w277] mode=indexing
              tunnel: [w276] -> w235 mode=indexing
              tunnel: [w275] -> w227
              n79 = Open/Create/Replace File(file path (use dialog)=w277, operation (0:open)=T10."replace or create", access (0:read/write)=enum16{"read/write", "read-only", "write-only"}."read/write", disable buffering (F)=TRUE) -> (refnum out=w276:refnum<file>, error out=w275:errorcluster)  [unwired: 1 in, 2 out]
            }
            n80 = xnode "Invoke Method"("FPGA VI Reference In"=w271, "error in"=w270, "Requested Depth"=w256) -> ("FPGA VI Reference Out"=w273:refnum<k20>, "error out"=w272:errorcluster)  [unwired: 1 out]
            n81 = Bundle By Name(cluster=w229, "Number of elements"=u32 0 ("Adquirir?"), "Time to Acquire Block (ms)"=w254, "Block Size"=w253, "Ref file Data"=w235) -> (w252:T3)
            n82 = xnode "Invoke Method"("FPGA VI Reference In"=w273, "error in"=w272) -> ("FPGA VI Reference Out"=w268:refnum<k20>, "error out"=w239:errorcluster)
            n83 = Merge Errors(w239, w227, w238, w234) -> (w237:errorcluster)
          }
          frame "Acquire and logging" {
            n84 = case shown="\"Idle\", Default" w296 {
              selector: w296 -> [w337 _]
              tunnel: w295 -> [w332 w379]
              tunnel: w294 -> [w304 w351]
              tunnel: w293 -> [w309 w362]
              tunnel: [w331 w370] -> w282
              tunnel: w287 -> [w312 w339]
              tunnel: [w337 w360] -> w291
              tunnel: w290 -> [_ w363]
              tunnel: [w304 w361] -> w289
              tunnel: [w308 w338] -> w288
              tunnel: w286 -> [w311 _]
              tunnel: [w302 w339] -> w285
              tunnel: w284 -> [w310 _]
              tunnel: w283 -> [w303 _]
              frame "Idle", Default {
                n85 = Unbundle By Name(w304) -> ("Buffer Overflow"=w300:bool, "Tiempo de paso (s)"=w328:dbl, "Nº Ruedas 1"=w301:i32, "NºRuedas 2"=w326:i32, "Ref file Data"=w325:refnum<file>[])
                n86 = Unbundle By Name(w312) -> ("Cfg.Direccion 0?"=w314:bool)
                n87 = xnode "Read/Write Control"("FPGA VI Reference In"=w332, "error in"=w309) -> ("FPGA VI Reference Out"=w333:refnum<k20>, "error out"=w298:errorcluster, "Chassis Temperature"=w329:i16)
                n88 = call "ErrorOverFlow.vi"("Buffer Overflow"=w300) -> ("error out"=w297:errorcluster)
                n89 = Multiply(x=w328, y=1000.0) -> (x*y=w317:dbl)
                n90 = Divide(x=w329, y=4.0) -> (x/y=w318:dbl)
                n91 = Bundle By Name(cluster=w312, "Cfg.Temperatura (ºC)"=w318) -> (w302:cluster{"File path":T4, "Cfg ":T5})
                n92 = Build Array(w318, w317, w301) -> (w316:dbl[])
                n93 = Build Array(w318, w317, w301, w326) -> (w323:dbl[])
                n94 = To Single Precision Float(number=w316) -> (single precision float=w315:sgl[])
                n95 = call "close data logs.vi"("error in"=w309, "Data"=w315, "Ref file Data"=w325) -> ("error out"=w322:errorcluster)  [unwired: 8 in]
                n96 = Merge Errors(w298, w297) -> (w299:errorcluster)
                n97 = call "send_multiple_queue.vi"("error in (no error)"=w309, "Processing"=w310, "RFID"=w311, "info"=w302) -> ("error out"=w313:errorcluster)  [unwired: 7 in]
                n98 = xnode "Read/Write Control"("FPGA VI Reference In"=w333, "error in"=w298, "Stop"=TRUE ("stop")) -> ("FPGA VI Reference Out"=w335:refnum<k20>, "error out"=w334:errorcluster)
                n99 = Bundle("error IO"=w299, w323, "Direccion 0?"=w314, "error out"=w322) -> (w319:T14)  [unwired: 1 in]
                n100 = xnode "Invoke Method"("FPGA VI Reference In"=w335, "error in"=w334) -> ("FPGA VI Reference Out"=w331:refnum<k20>, "error out"=w324:errorcluster)
                n101 = Merge Errors(w324, w322, w313) -> (w321:errorcluster)
                n102 = call-poly "Enqueue Message.vi"("error in (no error)"=w321, "Message Data"=w319, "Message"="Update Acq data", "Message Queue"=w303) -> ("error out"=w306:errorcluster, "dup Message Queue"=w307:refnum<queue>)  [unwired: 6 in]
                n103 = call-poly "Enqueue Message.vi"("error in (no error)"=w306, "Message Data"=w304, "Message"="Update test data", "Message Queue"=w307) -> ("error out"=w308:errorcluster)  [unwired: 6 in, 1 out]
              }
              frame "Acquiring" {
                # "logging"
                n104 = Unbundle By Name(w339) -> ("Cfg.Inicio pasada"=w354:timestamp, "Cfg.Tiempo extra al detector de paso (s)"=w359:dbl, "Cfg.Tiempo de adquisicion"=w355:dbl, "Cfg.Timeout ruedas"=w356:dbl)
                n105 = Unbundle By Name(w351) -> ("Number of elements"=w350:u32)
                n106 = xnode "Invoke Method"("FPGA VI Reference In"=w379, "error in"=w362, "Number of Elements"=w350, "Timeout (ms)"=0) -> ("FPGA VI Reference Out"=w378:refnum<k20>, "error out"=w373:errorcluster, "Data"=w375:fxp<+/-,24,4>[], "Elements Remaining"=w374:u32)
                n107 = Unbundle By Name(w351) -> ("Tiempo de paso (s)"=w352:dbl)
                n108 = call "log_data.vi"("error in (no error)"=w362, "Test"=w351, "Elements Remaining"=w374, "Data"=w375) -> ("error out"=w343:errorcluster, "Ref file Data out"=w366:refnum<file>[], "Number of elements out"=w365:u32)  [unwired: 5 in]
                n109 = xnode "Read/Write Control"("FPGA VI Reference In"=w378, "error in"=w373) -> ("FPGA VI Reference Out"=w376:refnum<k20>, "error out"=w372:errorcluster, "Parar"=w358:bool, "Nº Ruedas 1"=w368:i32, "NºRuedas 2"=w367:i32)
                n110 = xnode ("CheckLate")("FPGA VI Reference In"=w376, "error in"=w372) -> ("FPGA VI Reference Out"=w371:refnum<k20>, "error out"=w348:errorcluster, "Buffer Underflow"=w369:bool, "Buffer Overflow"=w349:bool)
                n111 = case shown="False" w358 {
                  tunnel: [w387 w394] -> w341
                  tunnel: [w382 0.0] -> w357
                  tunnel: w359 -> [_ w391]
                  tunnel: w355 -> [w383 _]
                  tunnel: w354 -> [w381 _]
                  tunnel: [w382 w390] -> w353
                  tunnel: w352 -> [_ w390]
                  frame False {
                    n112 = Get Date/Time In Seconds() -> (seconds since 1Jan1904=w388:timestamp)
                    n113 = local read "Adquirir manual"() -> (w380:bool)
                    n114 = To Double Precision Float(number=w388) -> (double precision float=w384:dbl)
                    "Tiempo" <- w384
                    n115 = To Double Precision Float(number=w381) -> (double precision float=w389:dbl)
                    n116 = Subtract(x=w384, y=w389) -> (x-y=w382:dbl)
                    n117 = Greater?(x=w382, y=w383) -> (0:w386:bool)
                    n118 = Select(t=w386, s=w380, f=FALSE) -> (s? t:f=w387:bool)
                  }
                  frame True {
                    n119 = local read "Tiempo"() -> (w392:dbl)
                    n120 = Get Date/Time In Seconds() -> (seconds since 1Jan1904=w395:timestamp)
                    n121 = To Double Precision Float(number=w395) -> (double precision float=w396:dbl)
                    n122 = Subtract(x=w396, y=w392) -> (x-y=w397:dbl)
                    n123 = Greater?(x=w397, y=w391) -> (0:w394:bool)
                  }
                }
                n124 = call-poly "Enqueue Message.vi"("error in (no error)"=w362, "Message"="Acquire and logging", "Message Queue"=w363) -> ("error out"=w338:errorcluster)  [unwired: 7 in, 1 out]
                n125 = call "ErrorOverFlow.vi"("Buffer Overflow"=w349) -> ("error out"=w347:errorcluster)
                n126 = Unbundle By Name(w343) -> ("status"=w342:bool)
                n127 = Merge Errors(w348, w347) -> (w346:errorcluster)
                n128 = Unbundle By Name(w346) -> ("status"=w345:bool)
                n129 = Greater?(x=w357, y=w356) -> (0:w340:bool)
                n130 = Bundle By Name(cluster=w351, "Buffer Underflow"=w369, "Buffer Overflow"=w349, "Nº Ruedas 1"=w368, "NºRuedas 2"=w367, "Number of elements"=w365, "Ref file Data"=w366, "Tiempo de paso (s)"=w353, "Timeout ruedas"=w340) -> (w361:T3)
                n131 = Compound Arithmetic op=OR(w345, w342, w341, w340) -> (w344:bool)
                n132 = case "Flush" shown="True" w344 {
                  tunnel: [w399 w405] -> _
                  tunnel: [w400 w404] -> w370
                  tunnel: w371 -> [w400 w403]
                  tunnel: w346 -> [w399 w402]
                  tunnel: [Acquisition_State."Acquiring" ("Acquisition State") Acquisition_State."Idle" ("Acquisition State")] -> w360
                  frame False {
                  }
                  frame True {
                    n133 = xnode "Invoke Method"("FPGA VI Reference In"=w403, "error in"=w402) -> ("FPGA VI Reference Out"=w404:refnum<k20>, "error out"=w405:errorcluster)
                  }
                }
              }
            }
          }
          frame "Reset" {
            w408 = FALSE ("Test")
            n134 = Bundle By Name(cluster=w410, "Test"=w408, "UPS"=w408, "Acquisicion"=w408, "Calibracion"=w408) -> (w409:T2)
            "Reset_controlador" <- TRUE ("Reset_controlador")
          }
          frame "Calibration" {
            n135 = Bundle By Name(cluster=w421, "Calibracion"=TRUE) -> (w420:T2)
          }
          frame "Start Acq Calibration" {
            w448 = "Calibration" ("element")
            w447 = "c"
            n136 = for {
              N: 1 -> [_]
              shift-right: [w460] -> w451
              shift-left: _ -> [w461]
              n137 = Add(x=w461, y=0.001) -> (x+y=w460:dbl)
            }
            n138 = Number To Fractional String(number=w451) -> (F-format string=w456:string)  [unwired: 3 out]
            n139 = Search and Replace String(input string=w456, search string="." ("replace string (\"\")")) -> (result string=w454:string)  [unwired: 1 in, 8 out]
            n140 = for {
              N: 3 -> [_]
              shift-right: [w465] -> w442
              shift-left: w454 -> [w463]
              n141 = Search and Replace String(input string=w463, search string="0", offset=4 ("offset (0)")) -> (result string=w465:string)  [unwired: 1 in, 7 out]
            }
            n142 = Format Date/Time String(time format string (%c)="%Y-%m-%d-%H-%M-%S") -> (date/time string=w441:string)  [unwired: 2 in]
            n143 = call-poly "Enqueue Message.vi"("error in (no error)"=w433, "Message"="Config calibration", "Message Queue"=w436) -> ("error out"=w430:errorcluster)  [unwired: 7 in, 1 out]
            n144 = Concatenate Strings(w442, "_" ("replace string (\"\")"), w441) -> (w443:string)
            n145 = Build Array(w447, w448, w443) -> (w446:string[])
            n146 = Build Array(w447, w448, w443, "Calibration_LOG.txt" ("element")) -> (w450:string[])
            n147 = Array of Strings to Path(0:w446) -> (2:w439:path)  [unwired: 1 out]
            n148 = Array of Strings to Path(0:w450) -> (2:w438:path)  [unwired: 1 out]
            n149 = Create Folder(path (use dialog)=w439) -> ()  [unwired: 2 in, 3 out]
            n150 = Bundle By Name(cluster=w427, "Archivo"=0.0) -> (w425:T1)
            n151 = Bundle By Name(cluster=w440, "File path.Folder calibration"=w439, "File path.calibration log"=w438) -> (w434:cluster{"File path":T4, "Cfg ":T5})
            n152 = call-poly "Enqueue Message.vi"("error in (no error)"=w433, "Message Data"=w434, "Message"="Update Settings", "Message Queue"=w435) -> ("error out"=w431:errorcluster)  [unwired: 6 in, 1 out]
            n153 = Merge Errors(w431, w430) -> (w432:errorcluster)
          }
          frame "Config calibration" {
            n154 = Unbundle By Name(w505) -> ("Cfg.Frecuencia de muestreo y módulo CRIO"=w504:T6, "Cfg.Count(mSec)"=w503:u32, "Cfg.Frecuencia de muestreo (Hz)"=w499:dbl, "Cfg.Escaneos de la FIFO por canal"=w498:u32, "Cfg.Nº de acelerómetros"=w501:i32, "Cfg.Nº inductivos"=w500:i32, "File path.Folder calibration"=w490:path)
            n155 = xnode "Invoke Method"("FPGA VI Reference In"=w522, "error in"=w467) -> ("FPGA VI Reference Out"=w507:refnum<k20>, "error out"=w518:errorcluster)  [unwired: 1 in]
            n156 = Unbundle By Name(w488) -> ("Archivo"=w509:dbl)
            n157 = Increment(x=w509) -> (x+1=w489:dbl)
            n158 = call "Time Delay"("error in (no error)"=w518, "Delay Time (s)"=1.0) -> ("error out"=w470:errorcluster)  [unwired: 9 in]
            n159 = Number To Decimal String(number=w489) -> (decimal integer string=w508:string)  [unwired: 1 in]
            n160 = Path to Array of Strings(0:w490) -> (2:w486:string[])  [unwired: 1 out]
            n161 = call "create calibration file name.vi"("Folder Calibraion"=w486) -> ("Name file"=w487:string[])  [unwired: 10 in]
            n162 = Concatenate Strings("\nAcquiring file: ", w508, "/11\n" ("string")) -> (w475:string)
            n163 = xnode "Read/Write Control"("FPGA VI Reference In"=w507, "error in"=w470, "Fotocélula"=TRUE ("Adquirir")) -> ("FPGA VI Reference Out"=w513:refnum<k20>, "error out"=w512:errorcluster)
            n164 = Array of Strings to Path(0:w487) -> (2:w477:path)  [unwired: 1 out]
            n165 = xnode "Read/Write Control"("FPGA VI Reference In"=w513, "error in"=w512, "Data Rate"=w504, "Digital?"=TRUE, "Count(mSec)"=w503) -> ("FPGA VI Reference Out"=w515:refnum<k20>, "error out"=w514:errorcluster)
            n166 = Add(x=w501, y=w500) -> (x+y=w497:i32)
            n167 = call-poly "Enqueue Message.vi"("error in (no error)"=w467, "Message"="Acq calibration", "Message Queue"=w491) -> ("error out"=w468:errorcluster)  [unwired: 7 in, 1 out]
            n168 = call "DMACalc.vi"("Number of Channels"=w497, "Number of Samples"=w498, "Rate (Hz)"=w499) -> ("Block Size"=w495:u32, "Time to Acquire Block (ms)"=w496:i32, "Host Buffer Size"=w502:u32)  [unwired: 6 in]
            n169 = xnode "Invoke Method"("FPGA VI Reference In"=w515, "error in"=w514, "Requested Depth"=w502) -> ("FPGA VI Reference Out"=w517:refnum<k20>, "error out"=w516:errorcluster)  [unwired: 1 out]
            n170 = Open/Create/Replace File(file path (use dialog)=w477, operation (0:open)=T10."replace or create", access (0:read/write)=enum16{"read/write", "read-only", "write-only"}."read/write", disable buffering (F)=TRUE) -> (refnum out=w482:refnum<file>)  [unwired: 1 in, 3 out]
            n171 = flat-sequence {
              tunnel: [w526] -> w493
              tunnel: w469 -> [_]
              frame #0 {
                n172 = Get Date/Time In Seconds() -> (seconds since 1Jan1904=w526:timestamp)
              }
            }
            n173 = Path To String(path=w477) -> (string=w479:string)
            n174 = xnode "Invoke Method"("FPGA VI Reference In"=w517, "error in"=w516) -> ("FPGA VI Reference Out"=w506:refnum<k20>, "error out"=w469:errorcluster)
            n175 = Concatenate Strings("\nFile created: ", w479, "\n", w475) -> (w474:string)
            n176 = Bundle By Name(cluster=w488, "Number of elements"=u32 0, "Time to Acquire Block (ms)"=w496, "Block Size"=w495, "Archivo"=w489, "Inicio pasada"=w493, "ref file"=w482) -> (w494:T1)
            n177 = call-poly "Enqueue Message.vi"("error in (no error)"=w467, "Message Data"=w474, "Message"="Update Status", "Message Queue"=w480) -> ("error out"=w472:errorcluster)  [unwired: 6 in, 1 out]
            n178 = Merge Errors(w469, w472, w468) -> (w473:errorcluster)
          }
          frame "Acq calibration" {
            n179 = case shown="\"Calibration_acq\"" w541 {
              selector: w541 -> [w546 _ _]
              tunnel: w540 -> [w545 w564 w617]
              tunnel: w538 -> [w544 w562 w581]
              tunnel: [w545 w563 w614] -> w537
              tunnel: w536 -> [w543 w547 w612]
              tunnel: [w543 w547 w611] -> w535
              tunnel: w534 -> [w542 w559 w586]
              tunnel: [w544 w562 w606] -> w533
              tunnel: [w546 Acquisition_State."Idle" ("Acquisition State") w588] -> w532
              tunnel: [w542 w556 w584] -> w531
              tunnel: w530 -> [_ w554 w585]
              tunnel: w529 -> [_ w560 _]
              tunnel: w527 -> [_ w553 _]
              frame "Idle", Default {
              }
              frame "Calibration" {
                n180 = Unbundle By Name(w562) -> ("Archivo"=w558:dbl, "error FPGA"=w570:errorcluster, "ref file"=w561:refnum<file>)
                n181 = call "Reporting_error.vi"("error out 2"=w570, "Concept"="FPGA ") -> ("Reporting"=w568:string)  [unwired: 1 in]
                n182 = Close File(refnum=w561, error in=w559) -> ()  [unwired: 2 out]
                n183 = xnode "Read/Write Control"("FPGA VI Reference In"=w564, "error in"=w559, "Stop"=TRUE) -> ("FPGA VI Reference Out"=w566:refnum<k20>, "error out"=w567:errorcluster)
                n184 = call-poly "Enqueue Message.vi"("error in (no error)"=w559, "Message Data"=w568, "Message"="Update Status", "Message Queue"=w560) -> ("error out"=w549:errorcluster, "dup Message Queue"=w550:refnum<queue>)  [unwired: 6 in]
                n185 = Greater?(x=w558, y=10.0) -> (0:w555:bool)
                n186 = xnode "Invoke Method"("FPGA VI Reference In"=w566, "error in"=w567) -> ("FPGA VI Reference Out"=w563:refnum<k20>)  [unwired: 1 out]
                n187 = call-poly "Enqueue Message.vi"("error in (no error)"=w549, "Message Data"=w547, "Message"="Update test data", "Message Queue"=w550) -> ("error out"=w548:errorcluster)  [unwired: 6 in, 1 out]
                n188 = case shown="False" w555 {
                  tunnel: w548 -> [w575 w579]
                  tunnel: [w574 w578] -> w556
                  tunnel: w554 -> [w573 _]
                  tunnel: w553 -> [_ w577]
                  frame False {
                    n189 = call-poly "Enqueue Message.vi"("error in (no error)"=w575, "Message"="Config calibration", "Message Queue"=w573) -> ("error out"=w574:errorcluster)  [unwired: 7 in, 1 out]
                  }
                  frame True {
                    n190 = call-poly "Enqueue Message.vi"("error in (no error)"=w579, "Message"="Acel_calib" ("Concept"), "Message Queue"=w577) -> ("error out"=w578:errorcluster)  [unwired: 7 in, 1 out]
                  }
                }
              }
              frame "Calibration_acq" {
                n191 = Unbundle By Name(w581) -> ("Number of elements"=w605:u32, "Inicio pasada"=w601:timestamp)
                n192 = Get Date/Time In Seconds() -> (seconds since 1Jan1904=w602:timestamp)
                n193 = xnode "Invoke Method"("FPGA VI Reference In"=w617, "error in"=w586, "Number of Elements"=w605, "Timeout (ms)"=0) -> ("FPGA VI Reference Out"=w616:refnum<k20>, "error out"=w608:errorcluster, "Data"=w610:fxp<+/-,24,4>[], "Elements Remaining"=w609:u32)
                n194 = To Double Precision Float(number=w602) -> (double precision float=w603:dbl)
                n195 = To Double Precision Float(number=w601) -> (double precision float=w604:dbl)
                n196 = Subtract(x=w603, y=w604) -> (x-y=w599:dbl)
                n197 = call-poly "Enqueue Message.vi"("error in (no error)"=w586, "Message"="Acq calibration", "Message Queue"=w585) -> ("error out"=w583:errorcluster)  [unwired: 7 in, 1 out]
                n198 = Greater?(x=w599, y=1.0 ("Tiempo de adquisición")) -> (0:w598:bool)
                n199 = call "log_data_calibration.vi"("Calibration"=w581, "error in (no error)"=w586, "Elements Remaining"=w609, "Data"=w610) -> ("number of elements out"=w607:u32, "error out"=w582:errorcluster)  [unwired: 5 in]
                n200 = xnode ("CheckLate")("FPGA VI Reference In"=w616, "error in"=w608) -> ("FPGA VI Reference Out"=w615:refnum<k20>, "error out"=w594:errorcluster, "Buffer Underflow"=w595:bool, "Buffer Overflow"=w596:bool)
                n201 = call "ErrorOverFlow.vi"("Buffer Overflow"=w596) -> ("error out"=w592:errorcluster)
                n202 = call "ErrorUnderFlow.vi"("Buffer Overflow"=w595) -> ("error out"=w593:errorcluster)
                n203 = Merge Errors(w594, w593, w592) -> (w590:errorcluster)
                n204 = Unbundle By Name(w582) -> ("status"=w597:bool)
                n205 = Unbundle By Name(w590) -> ("status"=w591:bool)
                n206 = Compound Arithmetic op=OR(w591, w598, w597) -> (w589:bool)
                n207 = Bundle By Name(cluster=w612, "Buffer Underflow"=w595, "Buffer Overflow"=w596) -> (w611:T3)
                n208 = case "Flush" shown="False" w589 {
                  tunnel: w615 -> [w619 w625]
                  tunnel: w590 -> [w620 w624]
                  tunnel: [w620 w623] -> w580
                  tunnel: [w619 w622] -> w614
                  tunnel: [Acquisition_State."Calibration_acq" ("Acquisition State") Acquisition_State."Calibration" ("Acquisition State")] -> w588
                  frame False {
                  }
                  frame True {
                    n209 = xnode "Invoke Method"("FPGA VI Reference In"=w625, "error in"=w624) -> ("FPGA VI Reference Out"=w622:refnum<k20>, "error out"=w623:errorcluster)
                  }
                }
                n210 = Bundle By Name(cluster=w581, "Number of elements"=w607, "error FPGA"=w580) -> (w606:T1)
                n211 = Merge Errors(w580, w582, w583) -> (w584:errorcluster)
              }
            }
          }
          frame "UPS" {
            n212 = node-c288() -> (w638:T11)  [unwired: 4 in]
            n213 = timed-loop {
              timing: w638 -> [_]
              timing-out: [_] -> w637
              tunnel: w636 -> [w648]
              tunnel: [w647] -> w635
              tunnel: [w646] -> w627
              tunnel: w634 -> [w640]
              stop <- w641 stop-if-true
              n214 = node-c288() -> ()  [unwired: 1 in, 1 out]
              n215 = xnode "Read/Write Control"("FPGA VI Reference In"=w648, "error in"=w640) -> ("FPGA VI Reference Out"=w647:refnum<k20>, "error out"=w646:errorcluster, "DC OK"=w644:bool, "Chassis Temperature"=w645:i16)
              n216 = call "ControlTemperatura.vi"("Chassis Temperature"=w645) -> ("T fuera rango"=w643:bool)  [unwired: 2 out]
              n217 = Not(x=w643) -> (.not. x?=w642:bool)
              n218 = And(x=w644, y=w642) -> (x .and. y?=w641:bool)
              n219 = node-c288() -> ()  [unwired: 1 in, 1 out]
            }
            n220 = node-c288(w637) -> ()  [unwired: 1 out]
            n221 = call-poly "Enqueue Message.vi"("error in (no error)"=w627, "Message"="Espera", "Message Queue"=w628) -> ("error out"=w629:errorcluster)  [unwired: 7 in, 1 out]
          }
          frame "Exit" {
            n222 = Release Queue(queue=w661, error in (no error)=w662) -> (error out=w659:errorcluster)  [unwired: 1 in, 2 out]
            n223 = xnode "Close FPGA VI Reference"("FPGA VI Reference In"=w657, "error in"=w659) -> ("error out"=w658:errorcluster)
          }
          frame Default {
            n224 = xnode "Error Ring"("parameter 0"=w669) -> ("error out"=w670:errorcluster)
          }
        }
      }
    }
    frame Error {
    }
  }
  "error out" <- w1
